vi "15-DuplicateInput(pt2).vi"(11 "Risk Array in":u8[][](array[numeric])) -> (3 "Risk Array out":u8[][](array[numeric]))   [LabVIEW 2019, in "15.lvlib"]
uses:
  15.lvlib
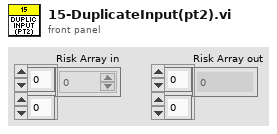
[diagram p1: front panel]
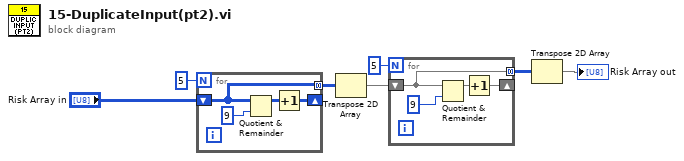
[diagram p0: block diagram]
diagram:
  n1 = for {
    N: 5 -> [_]
    shift-right: [w8] -> _
    shift-left: "Risk Array in" -> [w9]
    tunnel: [w9] -> w2 mode=concatenating
    n2 = Quotient & Remainder(x=w9, y=u8 9 ("String")) -> (x-y*floor(x/y)=w10:u8[][])  [unwired: 1 out]
    n3 = Increment(x=w10) -> (x+1=w8:u8[][])
  }
  n4 = Transpose 2D Array(2D array=w2) -> (transposed array=w3:u8[][])
  n5 = for {
    N: 5 -> [_]
    shift-right: [w12] -> _
    shift-left: w3 -> [w13]
    tunnel: [w13] -> w4 mode=concatenating
    n6 = Quotient & Remainder(x=w13, y=u8 9 ("String")) -> (x-y*floor(x/y)=w14:u8[][])  [unwired: 1 out]
    n7 = Increment(x=w14) -> (x+1=w12:u8[][])
  }
  n8 = Transpose 2D Array(2D array=w4) -> (transposed array=→"Risk Array out":u8[][])
